vi "ClassInVi.vi"() -> ()   [LabVIEW 2013]
uses:
  DebugClass.lvclass
panel:
  out "DebugClass.lvclass 2":refnum<class "DebugClass.lvclass">
  in  "DebugClass.lvclass":refnum<class "DebugClass.lvclass">
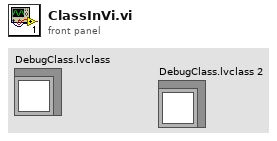
[diagram p1: front panel]
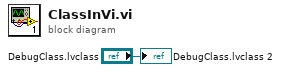
[diagram p0: block diagram]
diagram:
  "DebugClass.lvclass 2" <- "DebugClass.lvclass"
